vi "Test_WriteItemTwice_SameType_Replaced.vi"(8 "error in (no error)":errorcluster, 11 "TestCase in":refnum<class "TestComposedLookupTable.lvclass">) -> (0 "error out":errorcluster, 3 "TestCase out":refnum<class "TestComposedLookupTable.lvclass">)   [LabVIEW 2017, in "TestComposedLookupTable.lvclass"]
uses:
  TestComposedLookupTable.lvclass
  Source/LookupTable/LookupTable.lvclass/LookupTable.ctl
  795aeb50-7324-4620-a4ed-731e649c4fc8.vi
  0f4fd84d-09cb-4032-bd40-49a8e65684c7.vi
  Source/LookupTable/Read Table Reference.vi
  795aeb50-7324-4620-a4ed-731e649c4fc8.vi/b2b33031-2e50-4a66-972d-e6db33d63ec3.vi
  0f4fd84d-09cb-4032-bd40-49a8e65684c7.vi/875be668-9eca-4cd5-b873-efe56c1990f2.vi
  Source/LookupTable/LookupTable.lvclass
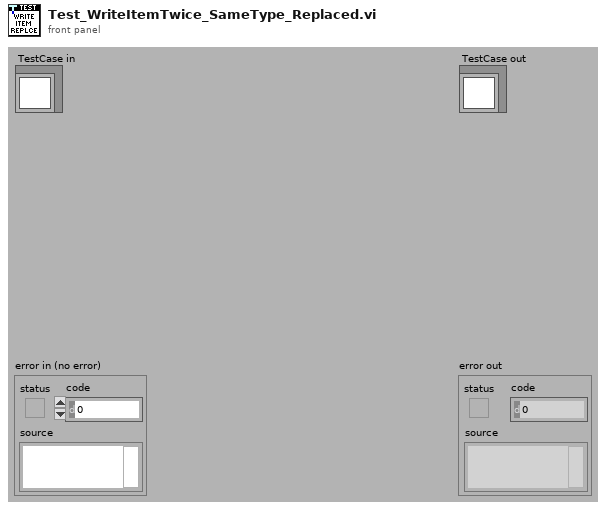
[diagram p1: front panel]
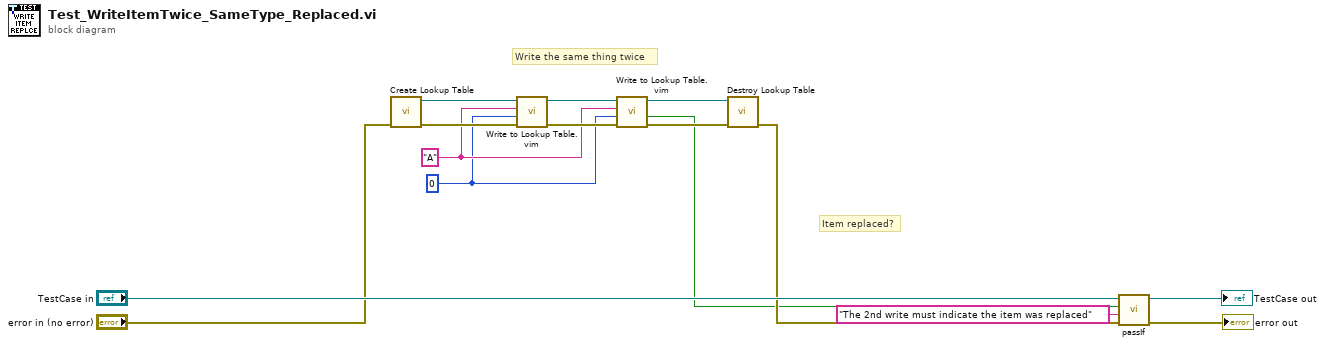
[diagram p0: block diagram]
diagram:
  w8 = 0
  w9 = "A" ("Item Name")
  # "Write the same thing twice"
  # "Item replaced?"
  n1 = call "Create Lookup Table.vi"("error in (no error)"="error in (no error)") -> ("error out"=w15:errorcluster, "LookupTable Reference"=w6:refnum<data-value>)  [unwired: 9 in]
  n2 = call "Write to Lookup Table.vim"("error in (no error)"=w15, "Item"=w8, "Item Name"=w9, "LookupTable Reference"=w6) -> ("error out"=w10:errorcluster, "LookupTable Reference Out"=w11:refnum<data-value>)  [unwired: 5 in, 1 out]
  n3 = call "Write to Lookup Table.vim"("error in (no error)"=w10, "Item"=w8, "Item Name"=w9, "LookupTable Reference"=w11) -> ("error out"=w3:errorcluster, "Replaced?"=w1:bool, "LookupTable Reference Out"=w4:refnum<data-value>)  [unwired: 5 in]
  n4 = call "Destroy Lookup Table.vi"("error in (no error)"=w3, "LookupTable Reference"=w4) -> ("error out"=w2:errorcluster)  [unwired: 9 in]
  n5 = call-dynamic "passIf.vi"("error in (no error)"=w2, "message (\"\")"="The 2nd write must indicate the item was replaced" ("message (\"\")"), "pass"=w1, "TestCase in"="TestCase in") -> ("error out"=→"error out":errorcluster, "TestCase out"=→"TestCase out":refnum<class "TestComposedLookupTable.lvclass">)  [unwired: 6 in]
